vi "PathPlanner_PathFinder_ClearG.vi"() -> (3 "G":map{i32, dbl}(c390))   [LabVIEW 2019]
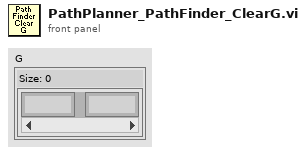
[diagram p1: front panel]
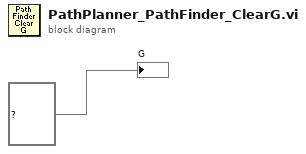
[diagram p0: block diagram]
diagram:
  "G" <- map{i32, dbl} {} ("G")
